vi "AlliGator Export Plugin Parameters to Clipboard.vi"(8 "Error In":errorcluster, 9 "Parameter Names only":bool, 11 "AlliGator IV DVR":refnum<data-value>) -> (0 "Error Out":errorcluster, 1 "Message":string, 3 "AlliGator IV DVR":refnum<data-value>)   [LabVIEW 2021, in "AlliGator Python Plugins.lvlib"]
doc: "Sends a string containing all parameters, internal variables and data accessible to python plugins."
uses:
  AlliGator Python Plugins.lvlib
  AlliGator Internal Variables v2.ctl
  <vilib>/vision/Image Controls.llb/IMAQ Image.ctl
  AlliGator Gate Image Set.ctl
  AlliGator FLI Dataset Type.ctl
  AlliGator Data Series Type.ctl
  AlliGator Dataset Channel.ctl
  AlliGator Gate Arithmetic.ctl
  AlliGator Displayed Image.ctl
  Image/Named ROI Description.ctl
  AlliGator Decay Metadata v3.ctl
  AlliGator Decay Background Subtraction Info.ctl
  AlliGator Baseline Subtraction Method.ctl
  Graphs/XY Graph/XY Graph Plot Shift Parameters.ctl
  Graphs/XY Graph/XY Graph Plot Shift Method.ctl
  AlliGator Decay Extrapolation Parameters.ctl
  Phasor/Calibration Phasor (m, phi).ctl
  Phasor/Phasor Reference Series.ctl
  Phasor/Phasor Calibration Map v2.ctl
  Phasor/Phasor (g, s).ctl
  AlliGator Raw Phasor Plot Data v4.ctl
  Phasor/Phasor Standard Deviation Options.ctl
  AlliGator Phasor Multi-Harmonic Data.ctl
  Phasor/Phasor Harmonic Data.ctl
  AlliGator Decay Fit Options & Parameters v2.ctl
  Fits/IRF(X)PSED/Decay Fit Options v2.ctl
  Fits/Decay Convolution/Decay Model.ctl
  Fits/Residual Type.ctl
  Fits/IRF(X)PSED/Fit Weights Type.ctl
  Fits/Non-linear Fitting Method v2.ctl
  Fits/Fit Calculation Method.ctl
  Fits/Non-linear Fitting Algorithm.ctl
  AlliGator Decay Fit Parameter Constraints 2.ctl
  Fits/IRF(X)PSED/Decay Fit Parameters In List.ctl
  Fits/IRF(X)PSED/MLE Baseline Offset Type.ctl
  AlliGator Decay Preprocessing Parameters.ctl
  Fits/IRF(X)PSED/Decay Fit Parameters & Derived Quantities List.ctl
  ec775fbe-273a-4088-92c5-d89fd97e82c2.vi
  ac933e2b-790f-40e3-b0ca-ca83e507d5bf.vi
  49bf73b8-9f3b-4d7e-9824-64ced49957da.vi
  <userlib>/_OpenG.lib/array/array.llb/Sort 1D Array (String)__ogtk.vi
  <userlib>/_OpenG.lib/array/array.llb/Reorder 1D Array2 (I32)__ogtk.vi
  <vilib>/JDP Science/JSONtext/Variant to JSON Text.vi
  <vilib>/JDP Science/JSONtext/LVClass Serializer/JSONtext LVClass Serializer.lvclass
  AlliGator Settings.lvlib
  Strings/Strings.lvlib
  AlliGator Globals, Variables & Constants.lvlib
  <userlib>/_OpenG.lib/array/array.llb/openg_array.lvlib
  Phasor/Phasor.lvlib
  Image/Image.lvlib
  AlliGator Decay Preprocessing.lvlib
  Graphs/XY Graph/XY Graph Add-Ons.lvlib
  AlliGator Phasor Graph.lvlib
  AlliGator Files.lvlib
  AlliGator Internal Variables.lvlib
  AlliGator Phasor Plot.lvlib
  AlliGator Source Image.lvlib
  Fits/Fits.lvlib
  AlliGator Decay Fit.lvlib
  AlliGator Decay Fit Parameter Map.lvlib
  AlliGator Dual-Channel Datasets.lvlib
panel:
  # "see the AlliGator License on the block diagram (Ctrl+E or Window:Show Block Diagram)"
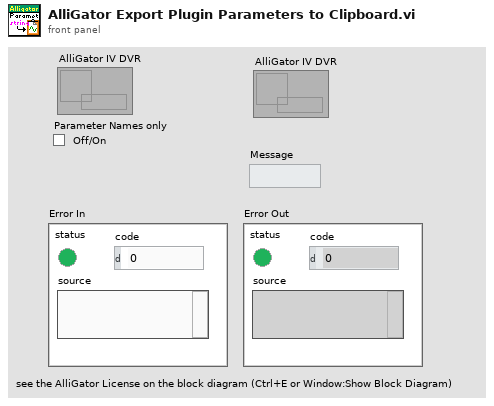
[diagram p1: front panel]
types:
  T1 = typedef "AlliGator Internal Variables.lvlib/AlliGator Internal Variables v2.ctl" = cluster{"Displayed Image":T2, "White Light Image":T2, "Mask Image":T2, "ROI Mask Image":T2, "Current Dataset Images 1":T3, "Background Dataset Images 1":T3, "Current Dataset Images 2":T3, "Background Dataset Images 2":T3, "Current Dataset Arithmetic Images":T3, "Accumulated Dataset Images 1":T3, "Accumulated Dataset Images 2":T3, "Accumulated Dataset Arithmetic Images":T3, "Phasor Plot Image":T2, "Decay Fit Parameter Map Image":T2, "Single Data Point Path":path, "White Light Image Path":path, "Mask Image Path":path, "Time-Series Folder":path, "[Time-Series Paths]":path[], "Current Dataset":i32, "Single Dataset Type":T4, "Current Folder":string, "AlliGator Data Series Type":T5, "# Datasets":i32, "Dual-Channel Dataset":bool, "Selected Channel Name":string, "Dataset Channel":T6, "Channel Arithmetic":T7, "Dual-Channel Background Dataset":bool, "Background Channel":T6, "Dual-Channel Accumulated Dataset":bool, "Start Time":dbl, "[Time-Series Timestamps]":dbl[], "[Intensity Corrections]":dbl[], "Time Series Script":bool, "Type of Displayed Image":T8, "Gate Image Slide":u16, "# Gates":i32, "ROIs":T9[], "ROI Decay":cluster{"t Array":dbl[], "I Array":dbl[]}, "Valid Decay":bool, "Decay  Metadata":T11, "Reference Decay Plot Name":string, "Reference Decay":cluster{"t Array":dbl[], "I Array":dbl[]}, "Decay Shift Plot":cluster{"Time Stamps":dbl[], "Decay Shifts":dbl[]}, "[Decays Max Values]":sgl[], "[Decays Min Values]":sgl[], "Calibration Phasor":T17, "Calibration Phasor Series":T18, "Phasor Calibration Map":T19, "Calibration Map MD5 Digest":string, "Last Raw Phasor":T20, "Last Calibrated Phasor":T20, "Last Calibrated Phasor SDV":T20, "Phasor Graph:Phasor Plot":cluster{"g Array":dbl[], "s Array":dbl[]}, "Phasor Graph:Phasor SDV Plot":cluster{"g Array":dbl[], "s Array":dbl[]}, "[Phasor Graph:Raw Phasor Plots]":T21[], "Phasor Plot locked to Ref 1":i32, "[Phasor Plot(s) locked to Ref 1]":i32[], "[Phasor Plot(s) locked to Ref 2]":i32[], "[Pixel Phasors]":T20[], "[[Sum Image]]":dbl[][], "[[CSG Phasors]]":csg[][], "[[Valid Pixel?]]":bool[][], "I/m/phi Dataset":cluster{"I/m/phi Dataset?":bool, "Base Frequency":dbl[unit], "Harmonic Orders":u8[]}, "Multi Phasor Plot Data":T23, "Decay Fit Options & Parameters":T25, "Fit Options: Decay Preprocessing Parameters":T36, "Fit Options: Reference Decay":cluster{"t Array":dbl[], "I Array":dbl[]}, "Is Full Image Parameters Map":bool, "Is Single-Pixels Parameters Map":bool, "NLSF Parameters Map X Resolution":i32, "NLSF Parameters Map Y Resolution":i32, "[Single Decay Fit Parameters]":dbl[], "Fit Model":T27, "[[Multiple Decays Fit Parameters]]":dbl[][], "[[Multiple Decays Fit Parameter SDVs]]":dbl[][], "[[IRFs]]":dbl[][], "IRF Array Time Axis":dbl[], "Decay Array Time Axis":dbl[], "[Decay Fit Parameter Names]":T37[], "[[Phasor Ratios]]":dbl[][], "[[Average Lifetimes]]":dbl[][], "Amplitude Weighted Average Lifetime":bool, "[Decay Sum]":dbl[], "[[User-defined Quantities]]":dbl[][], "User-defined Quantity":string}
  T2 = typedef "IMAQ Image.ctl" = refnum<image>
  T3 = typedef "AlliGator Internal Variables.lvlib/AlliGator Gate Image Set.ctl" = cluster{"SGL Image Max":T2, "SGL Image Sum":T2, "SGL Gate Images":T2[], "SGL Image Min":T2}
  T4 = typedef "AlliGator Files.lvlib/AlliGator FLI Dataset Type.ctl" = enum16{"HDF5 FLI Dataset", "Gate Image Folder", ".sdt FLI Dataset (Becker & Hickl)", ".ptu FLI Dataset (PicoQuant)", "SS1 FLI Dataset", "SS2 FLI Dataset", "I/m/phi Dataset", ".bin FLI Dataset (PicoQuant Binned)", ".bin FLI Dataset (Piccolo Binned)"}
  T5 = typedef "AlliGator Files.lvlib/AlliGator Data Series Type.ctl" = enum16{"Not a Supported Series", "Gate Images Folder Series", "SwissSPAD 2 Dataset Series", "B&H FLI Dataset Series", "PicoQuant PTU FLI Dataset Series", "PicoQuant BIN FLI Dataset Series", "Piccolo hist BIN FLI Dataset Series", "HDF5 FLI Dataset Series"}
  T6 = typedef "AlliGator Dual-Channel Datasets.lvlib/AlliGator Dataset Channel.ctl" = enum16{"G2", "INT"}
  T7 = typedef "AlliGator Settings.lvlib/AlliGator Gate Arithmetic.ctl" = enum16{"None", "INT-G2", "G2/INT*<INT>", "(1 - G2/INT)*<INT>"}
  T8 = typedef "AlliGator Source Image.lvlib/AlliGator Displayed Image.ctl" = enum16{"Single Gate", "Sum of All Gates", "Max of All Gates", "Min of All Gates", "-", "White Ligth Image", "Mask Image"}
  T9 = typedef "Image.lvlib/Named ROI Description.ctl" = cluster{"ROI Descriptor":T10, "ROI Name":string, "Overlay Color":u32}
  T10 = typedef "ROI Descriptor" = cluster{"Global Rectangle":i32[], "Contours":cluster{"ID":enum32{"External", "Internal"}, "Type":u32, "Coordinates":i32[]}[]}
  T11 = typedef "AlliGator Phasor Graph.lvlib/AlliGator Decay Metadata v3.ctl" = cluster{"ROI Descriptor":T10, "ROI Center":cluster{"X":i32, "Y":i32}, "Decay Background Subtraction Info":T12, "Decay Reverted":bool, "Decay Smoothened":bool, "Decay Straightened":bool, "Fitted Tau (Decay Straightening)":dbl, "Decay Shift Parameters":T14, "Decay Shifted":bool, "Decay Extrapolated":bool, "Decay Extrapolation Parameters":T16, "Decay Normalized":bool, "Fold Decay":bool, "# Folds":u32}
  T12 = typedef "AlliGator Decay Analysis.lvlib/AlliGator Decay Preprocessing.lvlib/AlliGator Decay Background Subtraction Info.ctl" = cluster{"Laser Period":dbl[unit], "Gate Duration":dbl[unit], "Baseline Subtraction Method":T13, "Background Definition Range":cluster{"Min Gate":dbl[unit], "Max Gate":dbl[unit]}, "Total Intensity w/o Bkgd Subtraction":dbl, "Bkgd-subtracted Intensity (exp)":dbl, "# Data Points":i32, "Background/Gate":dbl, "Fitted Lifetime":dbl[unit], "Bkgd-subtracted Intensity (theo)":dbl}
  T13 = typedef "AlliGator Decay Analysis.lvlib/AlliGator Decay Preprocessing.lvlib/AlliGator Baseline Subtraction Method.ctl" = enum16{"Mean", "Min", "Square Gated Single-Exponential", "File", "Constant"}
  T14 = typedef "XY Graph Add-Ons.lvlib/XY Graph Plot Shift Parameters.ctl" = cluster{"Type":T15, "Shift":dbl[unit], "Threshold":dbl, "Rotate":bool}
  T15 = typedef "XY Graph Add-Ons.lvlib/XY Graph Plot Shift Method.ctl" = enum16{"Default", "CFD", "Threshold", "Cross-Correlation"}
  T16 = typedef "AlliGator Decay Analysis.lvlib/AlliGator Decay Preprocessing.lvlib/AlliGator Decay Extrapolation Parameters.ctl" = cluster{"Additional Points":u32, "Head Fraction":dbl, "Fitted Tau":dbl, "Use Periodicity":bool, "Use Cursors":bool, "Tail Fraction":dbl}
  T17 = typedef "Phasor.lvlib/Calibration Phasor (m, phi).ctl" = cluster{"m":dbl, "phi":dbl, "Phasor Frequency":dbl[unit], "Reference Lifetime":dbl[unit]}
  T18 = typedef "Phasor.lvlib/Phasor Reference Series.ctl" = cluster{"m Array":dbl[], "phi Array":dbl[], "Phasor Frequency":dbl[unit], "Calibration Lifetime":dbl[unit]}
  T19 = typedef "Phasor.lvlib/Phasor Calibration Map v2.ctl" = cluster{"Phasor Frequency":dbl[unit], "Calibration Lifetime":dbl[unit], "ROI Centers":cluster{"X":i32, "Y":i32}[], "ROI Descriptors":T10[], "Map Resolution X":i32, "Map Resolution Y":i32, "z Array":cdb[]}
  T20 = typedef "Phasor.lvlib/Phasor (g, s).ctl" = cluster{"g":dbl, "s":dbl}
  T21 = typedef "AlliGator Phasor Graph.lvlib/AlliGator Raw Phasor Plot Data v4.ctl" = cluster{"Phasor Plot Name":string, "Raw Phasor Plot":T20[], "Phasor Frequency":dbl[unit], "[Decay Metadata]":T11[], "Raw Phasor Plot SDV":T20[], "Phasor SDV Options":T22, "[Calibration Phasor]":T17[]}
  T22 = typedef "Phasor.lvlib/Phasor Standard Deviation Options.ctl" = cluster{"Compute Estimated SDV":bool, "# Replicas":u32, "Use Estimated Average Phasor":bool}
  T23 = typedef "AlliGator Phasor Plot.lvlib/AlliGator Phasor Multi-Harmonic Data.ctl" = cluster{"Base Frequency":dbl[unit], "# Harmonics":u8, "Harmonic Orders":u8[], "Phasor Plot Settings Checksum":u64, "Phasor Harmonic Data Array":T24[]}
  T24 = typedef "Phasor.lvlib/Phasor Harmonic Data.ctl" = cluster{"Phasor Harmonic Name":string, "Phasor Plot Settings Checksum":u64, "Phasor Frequency":dbl[unit], "Base Frequency":dbl[unit], "Harmonic Order":u8, "Phasor Plot Parameters":string, "Phasor Array [[CSG]]":csg[][], "Dataset File Path":path}
  T25 = typedef "AlliGator Decay Fit Parameter Map.lvlib/AlliGator Decay Fit Options & Parameters v2.ctl" = cluster{"SYNC Period":dbl[unit], "Fit Options":T26, "Fit Parameter Constraints":T33[], "MLE Baseline Offset":dbl, "MLE Baseline Offset Type":T35}
  T26 = typedef "Fits.lvlib/Decay Fit Options v2.ctl" = cluster{"Show Fit Residuals":bool, "Fit Model":T27, "Residual Type":T28, "Max Decay Percentile":dbl, "Min Decay Percentile":dbl, "Show Full Decay":bool, "Weights":T29, "Fitting Method":T30, "Compute Parameter Uncertainties":bool, "Periodic Boundaries":bool, "Model Calculation":T31, "Period":dbl[unit], "Termination Criteria":cluster{"Max Iterations":i32, "Max Function Calls":i32, "Max Time":dbl[unit], "Function Tolerance":dbl, "Parameter Tolerance":dbl, "Gradient Tolerance":dbl, "Min Lambda":dbl, "Max Lambda":dbl, "Initial Tick Count":u32}, "Offset Resolution":dbl[unit], "Use Local IRF":bool, "Fitting Algorithm":T32}
  T27 = typedef "Fits.lvlib/Decay Model.ctl" = enum16{"1-Exponential", "2-Exponentials"}
  T28 = typedef "Fits.lvlib/Residual Type.ctl" = enum16{"Standard", "Normalized", "Reduced"}
  T29 = typedef "Fits.lvlib/Fit Weights Type.ctl" = enum16{"Unweighted", "1/Variance", "Best of All"}
  T30 = typedef "Fits.lvlib/Non-linear Fitting Method v2.ctl" = enum16{"Least Square", "Least Absolute Residual", "Bisquare", "MLE", "-", "Best of All"}
  T31 = typedef "Fits.lvlib/Fit Calculation Method.ctl" = enum16{"Simulation", "Convolution", "Integration"}
  T32 = typedef "Fits.lvlib/Non-linear Fitting Algorithm.ctl" = enum16{"Levenberg-Marquardt", "Trust-Region Dogleg"}
  T33 = typedef "AlliGator Decay Analysis.lvlib/AlliGator Decay Fit.lvlib/AlliGator Decay Fit Parameter Constraints 2.ctl" = cluster{"Fit Parameter":T34, "Min Value":dbl, "Max Value":dbl, "Global":bool, "Used":bool}
  T34 = typedef "Fits.lvlib/Decay Fit Parameters In List.ctl" = enum16{"Offset", "Baseline", "A_1", "tau_1", "A_2", "tau_2"}
  T35 = typedef "Fits.lvlib/MLE Baseline Offset Type.ctl" = enum32{"Absolute", "Percentage"}
  T36 = typedef "AlliGator Decay Analysis.lvlib/AlliGator Decay Preprocessing.lvlib/AlliGator Decay Preprocessing Parameters.ctl" = cluster{"Background Subtraction":bool, "Straighten Decay":bool, "Reverse Gates":bool, "1-Normalized Decay":bool, "Smoothen Decay":bool, "Smoothing Parameter":dbl, "Shift Decay":bool, "Decay Shift Parameters":T14, "Extrapolate Decay":bool, "Additional Points":u32, "Head Fraction":dbl, "Pixel-Normalize Decay":bool, "Use Periodicity":bool, "Use Cursors":bool, "Tail Fraction":dbl, "Use Decay Pre-Processing":bool, "Fold Decay":bool, "# Folds":u32, "[0-1]-Normalized Decay":bool}
  T37 = typedef "Fits.lvlib/Decay Fit Parameters & Derived Quantities List.ctl" = enum16{"Offset", "Baseline", "A_1", "tau_1", "A_2", "tau_2", "<tau>_a", "f1_a", "f2_a", "<tau>_i", "f1_i", "f2_i", "-", "R^2", "Chi^2"}
  T38 = typedef "AlliGator Settings.lvlib/AlliGator Settings List.ctl" = enum16{"GUI:Visible Settings Tab", "GUI:Last Run Version", "Source Image:Use Image Histogram for Contrast", "Source Image:Low Count Pixels Rejection Options", "Source Image:High Count Pixels Rejection Options", "Source Image:Use Image Brightness", "Source Image:Blend Overlay with Image Background", "Source Image:Use Fixed ROI Diameter", "Source Image:ROI Diameter", "Source Image:ROI Center Color", "Source Image:Peak Threshold", "Source Image:Intensity Threshold", "Source Image:Image Binning Options", "Source Image:Image Smoothing Options", "Source Image:Image Histogram Active", "Source Image:Invert Binary Mask", "Source Image:Hot Pixel Removal", "Source Image:Overlay Analyzed ROI Center", "Source Image:Auto-Adjust Contrast", "Source Image:Histogram Lower Percentile", "Source Image:Histogram Upper Percentile", "Source Image:Save Source Image", "Source Image:Scale Bar Options", "Source Image:Image Resolution (Pixel Size)", "Source Image:Flatfield Correction", "Source Image:Show Dead Left Columns Correction", "Source Image:Dead Left Columns Correction", "Source Image:Image Pre-Processing Operations Order", "Data Information:Gate Width", "Data Information:Nanotime Gate Separation", "Data Information:Macrotime Gate Separation", "Data Information:Gate Step", "Data Information:# Gates", "Data Information:Gate Image Exposure", "Data Information:Gate Image Integration", "Data Information:Gates to Skip", "Data Information:Gates to Keep", "Data Information:Define Gates to", "Data Information:Channel Name", "Data Information:Available Channel Names", "Data Information:Channel Arithmetic", "Data Information:Background File Subtraction", "Data Information:Background File", "Data Information:Background Scaling Factor", "Data Information:Background Pile-up Correction", "Data Information:Background Pixel Well Capacity", "Data Information:Laser Period", "Data Information:SYNC Period", "Data Information:Pile-up Correction", "Data Information:Pixel Well Capacity", "Data Information:Dataset Scaling Factor", "Fluorescence Decay_Decay Pre-Processing:Reverse Gates", "Fluorescence Decay_Decay Pre-Processing:Verbose Decay Pre-Processing", "Fluorescence Decay_Decay Pre-Processing:Use Decay Pre-Processing", "Fluorescence Decay_Decay Pre-Processing:Background Subtraction", "Fluorescence Decay_Decay Pre-Processing:Background Definition Range", "Fluorescence Decay_Decay Pre-Processing:Baseline Subtraction Method", "Fluorescence Decay_Decay Pre-Processing:Decay Pre-Processing Operations Order", "Fluorescence Decay_Decay Pre-Processing:Smoothing Parameter", "Fluorescence Decay_Decay Pre-Processing:Shift Decay", "Fluorescence Decay_Decay Pre-Processing:Decay Shift Parameters", "Fluorescence Decay_Decay Pre-Processing:Fold Decay", "Fluorescence Decay_Decay Pre-Processing:# Folds", "Fluorescence Decay_Decay Pre-Processing:1-Normalize Decay", "Fluorescence Decay_Decay Pre-Processing:[0-1]-Normalize Decay", "Fluorescence Decay_Decay Pre-Processing:Smoothen Decay", "Fluorescence Decay_Decay Pre-Processing:Extrapolate Decay", "Fluorescence Decay_Decay Pre-Processing:Use Periodicity", "Fluorescence Decay_Decay Pre-Processing:Use Cursors", "Fluorescence Decay_Decay Pre-Processing:Tail Fraction", "Fluorescence Decay_Decay Pre-Processing:Head Fraction", "Fluorescence Decay_Decay Pre-Processing:Additional Points", "Fluorescence Decay_Decay Pre-Processing:Straighten Decay", "Fluorescence Decay_Decay Pre-Processing:Constant Background", "Fluorescence Decay_Decay Pre-Processing:Pixel-Normalize Decay", "Fluorescence Decay_Advanced Analysis:Extract IRF instead of Decay", "Fluorescence Decay_Advanced Analysis:IRF Extraction Options", "Fluorescence Decay_Advanced Analysis:IRF Optimization Options", "Fluorescence Decay_Advanced Analysis:Square Pulse Options", "Fluorescence Decay_Advanced Analysis:IRF Order", "Fluorescence Decay_Advanced Analysis:IRF Time Constants", "Fluorescence Decay_Advanced Analysis:Wavelet Analysis Options", "Fluorescence Decay_Advanced Analysis:Average Lifetime Options", "Fluorescence Decay_Fit Options:Fit Options", "Fluorescence Decay_Fit Options:Use Legacy Fitting Approach", "Fluorescence Decay_Fit Options:Use Data Information Laser Period", "Fluorescence Decay_Fit Parameters:Displayed Fit Parameters", "Fluorescence Decay_Fit Parameters:Fit Parameter Constraints", "Fluorescence Decay_Fit Parameters:Export Tabulated Results", "Fluorescence Decay_Fit Parameters:MLE Baseline Offset Type", "Fluorescence Decay_Fit Parameters:MLE Baseline Offset", "Fluorescence Decay_Fit Parameters:Guess Parameter Names", "Fluorescence Decay_Fit Parameters:Guess Parameter Values", "Fluorescence Decay_Fit Parameters:Guess Parameters Options", "Fluorescence Decay_Styles:Show Last Decay Only", "Fluorescence Decay_Styles:Decay Graph Color Array", "Fluorescence Decay:Decay Graph Active", "Fluorescence Decay Statistics:Min Peak Value", "Fluorescence Decay Statistics:Reject Low Decay Peak Pixels", "Fluorescence Decay Statistics:Reject High Decay Peak Pixels", "Fluorescence Decay Statistics:Max Peak Value", "Time Traces:Use File Timestamp", "Time Traces:Time Step", "Time Traces:Use Intensity Correction File", "Time Traces:Intensity Correction File", "Phasor Plot:Phasor Plot Smoothing Options", "Phasor Plot:Phasor Plot Size", "Phasor Plot:Phasor Plot Graphics Options", "Phasor Plot:Cumulative Phasor Plot", "Phasor Plot:Use Phasor Brightness", "Phasor Plot:Blend Overlay with Phasor Background", "Phasor Plot:Save Phasor Plot", "Phasor Plot:Show References", "Phasor Plot:Phasor Ratio Decay Range", "Phasor Plot:Exponential Fading", "Phasor Plot:Phasor Ratio Reference Colors", "Phasor Plot:Reference Radius", "Phasor Plot:Show Color Map Vertices", "Phasor Plot:Phasor Plot Active", "Phasor Plot:Phasor Ratio Color Map Type", "Phasor Plot:Phasor Ratio Color Map", "Phasor Plot:Phasor Ratio Display Range", "Phasor Plot:Selected Image ROI(s)", "Phasor Plot:All Image ROIs", "Phasor Plot:Selected Phasor Plot ROI(s)", "Phasor Plot:All Phasor Plot ROIs", "Phasor Plot:Phasor Ratio Color-Coded Quantity", "Phasor Plot:Store Phasor Harmonics", "Phasor Plot:Draw Reference Segment", "Phasor Plot:User-Defined Quantity", "Phasor Graph:Phasor Frequency", "Phasor Graph:Phasor Ratio Type", "Phasor Graph:Pixel-level Phasor Computation", "Phasor Graph:Save Phasor Graph", "Phasor Graph:Phasor Graph Active", "Phasor Graph:Phasor SDV Options", "Phasor Calibration:Use Backup Calibration if needed", "Phasor Graph:Define Shortest Lifetime as", "Phasor Calibration:Backup Calibration Type", "Phasor Calibration:Calibration Type", "Phasor Calibration:Calibration Lifetime", "Phasor Calibration:Calibration Map Algorithm", "Single-Exponential Phasor Locus (SEPL):Gate Parameters", "Single-Exponential Phasor Locus (SEPL):User-defined Gate", "Single-Exponential Phasor Locus (SEPL):User-defined IRF", "Single-Exponential Phasor Locus (SEPL):Phasor Parameters", "Single-Exponential Phasor Locus (SEPL):Decay & IRF Parameters", "Single-Exponential Phasor Locus (SEPL):Display Parameters", "Lifetime Analysis:Decay Analysis Parameters", "Lifetime Analysis:Lifetime Map Active", "Plugins:Python Settings", "Miscellaneous:Verbose Mode", "Miscellaneous:Beep after Script", "Miscellaneous:Saved Image File Format", "Miscellaneous:Exported Gate Image Settings", "Miscellaneous:Include Loading in Timing", "Miscellaneous:Verbose Settings Mode", "Miscellaneous:Histogram Options", "Miscellaneous:Beep on Error", "Miscellaneous:# Logical Processors Used", "Miscellaneous:ROI Description Max Characters", "Miscellaneous:Verbose Error Mode", "Miscellaneous:Transparent Mask Color"}
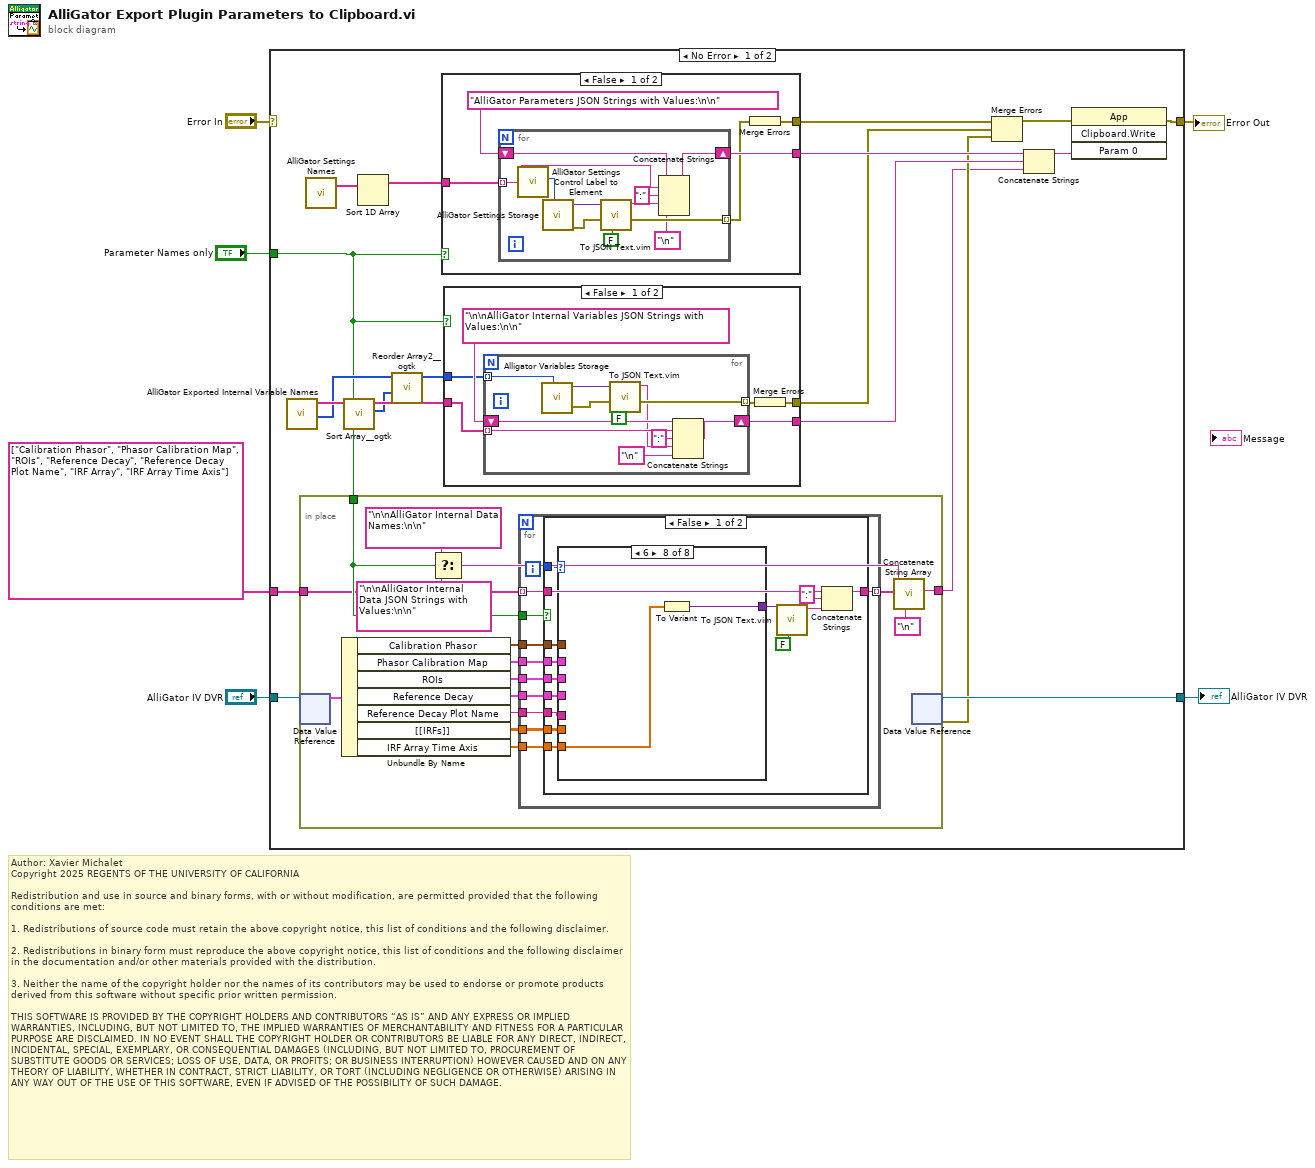
[diagram p0: block diagram]
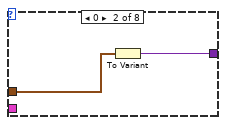
[diagram p3: hidden frame]
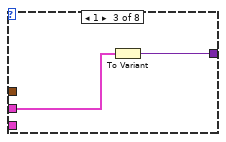
[diagram p4: hidden frame]
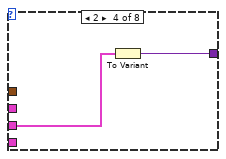
[diagram p5: hidden frame]
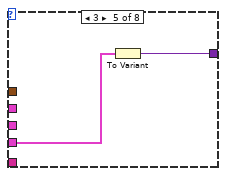
[diagram p6: hidden frame]
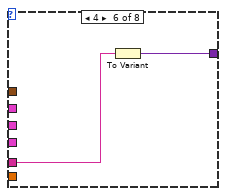
[diagram p7: hidden frame]
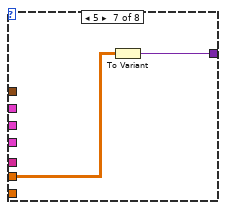
[diagram p8: hidden frame]
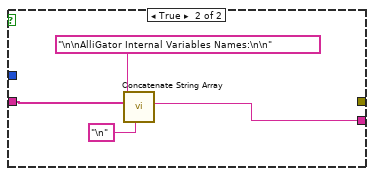
[diagram p10: hidden frame]
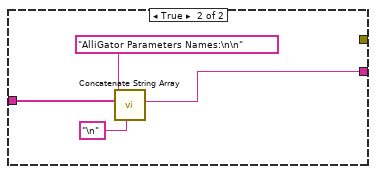
[diagram p11: hidden frame]
diagram:
  # "Author: Xavier Michalet\nCopyright 2025 REGENTS OF THE UNIVERSITY OF CALIFORNIA\n\nRedistribution and use in source and binary forms, with or without modification, are permitted provided that the following conditions are met:\n\n1. Redistributions of source code must retain the above copyright notice, this list of conditions and the following disclaimer.\n\n2. Redistributions in binary form must reproduce the above copyright notice, this list of conditions and the following disclaimer in the documentation and/or other materials provided with the distribution.\n\n3. Neither the name of the copyright holder nor the names of its contributors may be used to endorse or promote products derived from this software without specific prior written permission.\n\nTHIS SOFTWARE IS PROVIDED BY THE COPYRIGHT HOLDERS AND CONTRIBUTORS “AS IS” AND ANY EXPRESS OR IMPLIED WARRANTIES, INCLUDING, BUT NOT LIMITED TO, THE IMPLIED WARRANTIES OF MERCHANTABILITY AND FITNESS FOR A PARTICULAR PURPOSE ARE DISCLAIMED. IN NO EVENT SHALL THE COPYRIGHT HOLDER OR CONTRIBUTORS BE LIABLE FOR ANY DIRECT, INDIRECT, INCIDENTAL, SPECIAL, EXEMPLARY, OR CONSEQUENTIAL DAMAGES (INCLUDING, BUT NOT LIMITED TO, PROCUREMENT OF SUBSTITUTE GOODS OR SERVICES; LOSS OF USE, DATA, OR PROFITS; OR BUSINESS INTERRUPTION) HOWEVER CAUSED AND ON ANY THEORY OF LIABILITY, WHETHER IN CONTRACT, STRICT LIABILITY, OR TORT (INCLUDING NEGLIGENCE OR OTHERWISE) ARISING IN ANY WAY OUT OF THE USE OF THIS SOFTWARE, EVEN IF ADVISED OF THE POSSIBILITY OF SUCH DAMAGE."
  n1 = case shown="No Error" "Error In" {
    selector: "Error In" -> [_ w125]
    tunnel: "Parameter Names only" -> [w11 _]
    tunnel: [w15 w125] -> w5
    tunnel: "AlliGator IV DVR" -> [w14 w124]
    tunnel: [w13 w124] -> w2
    tunnel: string[] ["Calibration Phasor", "Phasor Calibration Map", "ROIs", "Reference Decay", "Reference Decay Plot Name", "IRF Array", "IRF Array Time Axis"] ("<JSON>") -> [w10 _]
    frame No Error {
      n2 = call "AlliGator Exported Internal Variable Names.vi"() -> ("Indices of Exported IVs"=w19:i32[], "Exported IV Name Array"=w24:string[])  [unwired: 10 in]
      n3 = in-place {
        in-place-border: w11 -> [w41]
        in-place-border: w10 -> [w40]
        in-place-border: [w39] -> w9
        n4 = in-place-dvr #1(w14) -> (w42:T1)  [unwired: 1 out]
        n5 = Unbundle By Name(w42) -> ("Calibration Phasor"=w38:T17, "Phasor Calibration Map"=w37:T19, "ROIs"=w36:T9[], "Reference Decay"=w35:cluster{"t Array":dbl[], "I Array":dbl[]}, "Reference Decay Plot Name"=w34:string, "[[IRFs]]"=w33:dbl[][], "IRF Array Time Axis"=w32:dbl[])
        n6 = Select(t="\n\nAlliGator Internal Data Names:\n\n", s=w41, f="\n\nAlliGator Internal Data JSON Strings with Values:\n\n") -> (s? t:f=w28:string)
        n7 = for {
          tunnel: w38 -> [w53]
          tunnel: w37 -> [w52]
          tunnel: w36 -> [w51]
          tunnel: w35 -> [w50]
          tunnel: w34 -> [w49]
          tunnel: w33 -> [w48]
          tunnel: w32 -> [w47]
          tunnel: [w46] -> w31 mode=indexing
          tunnel: w41 -> [w45]
          tunnel: w40 -> [w44] mode=indexing
          i -> [w43]
          n8 = case shown="False" w45 {
            tunnel: w53 -> [w67 _]
            tunnel: w52 -> [w66 _]
            tunnel: w51 -> [w65 _]
            tunnel: w50 -> [w64 _]
            tunnel: w49 -> [w63 _]
            tunnel: w48 -> [w62 _]
            tunnel: w47 -> [w61 _]
            tunnel: [w54 w82] -> w46
            tunnel: w44 -> [w56 w82]
            tunnel: w43 -> [w59 _]
            frame False {
              n9 = case shown="6" w59 {
                tunnel: w67 -> [_ w69 _ _ _ _ _ _]
                tunnel: w66 -> [_ _ w70 _ _ _ _ _]
                tunnel: w65 -> [_ _ _ w72 _ _ _ _]
                tunnel: w64 -> [_ _ _ _ w74 _ _ _]
                tunnel: w63 -> [_ _ _ _ _ w76 _ _]
                tunnel: w62 -> [_ _ _ _ _ _ w78 _]
                tunnel: w61 -> [_ _ _ _ _ _ _ w80]
                tunnel: [_ w68 w71 w73 w75 w77 w79 w81] -> w60
                frame -1, Default {
                }
                frame 0 {
                  n10 = To Variant(anything=w69) -> (Variant=w68:variant)
                }
                frame 1 {
                  n11 = To Variant(anything=w70) -> (Variant=w71:variant)
                }
                frame 2 {
                  n12 = To Variant(anything=w72) -> (Variant=w73:variant)
                }
                frame 3 {
                  n13 = To Variant(anything=w74) -> (Variant=w75:variant)
                }
                frame 4 {
                  n14 = To Variant(anything=w76) -> (Variant=w77:variant)
                }
                frame 5 {
                  n15 = To Variant(anything=w78) -> (Variant=w79:variant)
                }
                frame 6 {
                  n16 = To Variant(anything=w80) -> (Variant=w81:variant)
                }
              }
              n17 = call "To JSON Text.vim"("Pretty Print?"=FALSE, "Anything"=w60) -> ("<JSON>"=w57:string)  [unwired: 8 in, 1 out]
              n18 = Concatenate Strings(w56, ":" ("string"), w57) -> (w54:string)
            }
            frame True {
            }
          }
        }
        n19 = call "Concatenate String Array.vi"("Separator (TAB)"="\n", "String Array"=w31, "Prefix (\"\")"=w28) -> ("Formatted String"=w39:string)  [unwired: 8 in]
        n20 = in-place-dvr #1() -> (w13:refnum<data-value>, w12:errorcluster)  [unwired: 1 in]
      }
      n21 = call "AlliGator Settings Names.vi"() -> ("Settings Name Array"=w8:string[])  [unwired: 2 in, 1 out]
      n22 = call-poly <userlib>:"Sort Array__ogtk.vi"("Array in"=w24) -> ("Sorted Pointers"=w20:i32[], "Sorted Array out"=w23:string[])  [unwired: 9 in]
      n23 = Sort 1D Array(array=w8) -> (sorted array=w7:string[])
      n24 = call-poly <userlib>:"Reorder Array2__ogtk.vi"("indices"=w20, "array"=w19) -> ("reordered array"=w18:i32[])  [unwired: 9 in]
      n25 = case shown="False" w11 {
        tunnel: w7 -> [w108 w123]
        tunnel: [w107 w121] -> w25
        tunnel: [w105 _] -> w26
        frame False {
          n26 = for {
            tunnel: w108 -> [w111] mode=indexing
            shift-right: [w109] -> w107
            shift-left: "AlliGator Parameters JSON Strings with Values:\n\n" -> [w110]
            tunnel: [w113] -> w106 mode=indexing
            n27 = call "AlliGator Settings Control Label to Element.vi"("Control Label"=w111) -> ("AlliGator Settings List Element"=w119:T38)  [unwired: 7 in, 1 out]
            n28 = call "AlliGator Settings Storage.vi"("AlliGator Settings List"=w119) -> ("Error Out"=w117:errorcluster, "Variant Data out"=w118:variant)  [unwired: 9 in]
            n29 = call "To JSON Text.vim"("Pretty Print?"=FALSE, "error in (no error)"=w117, "Anything"=w118) -> ("error out"=w113:errorcluster, "<JSON>"=w115:string)  [unwired: 7 in]
            n30 = Concatenate Strings(w110, w111, ":" ("string"), w115, "\n" ("string")) -> (w109:string)
          }
          n31 = Merge Errors(w106) -> (w105:errorcluster)
        }
        frame True {
          n32 = call "Concatenate String Array.vi"("Separator (TAB)"="\n", "String Array"=w123, "Prefix (\"\")"="AlliGator Parameters Names:\n\n") -> ("Formatted String"=w121:string)  [unwired: 8 in]
        }
      }
      n33 = case shown="False" w11 {
        tunnel: w23 -> [w88 w102]
        tunnel: [w86 w100] -> w21
        tunnel: w18 -> [w85 _]
        tunnel: [w83 _] -> w16
        frame False {
          n34 = for {
            tunnel: w88 -> [w91] mode=indexing
            shift-right: [w92] -> w86
            shift-left: "\n\nAlliGator Internal Variables JSON Strings with Values:\n\n" -> [w93]
            tunnel: w85 -> [w99] mode=indexing
            tunnel: [w96] -> w84 mode=indexing
            n35 = call "Alligator Variables Storage.vi"("AlliGator Variable"=w99) -> ("Error Out"=w97:errorcluster, "Data out"=w98:variant)  [unwired: 8 in, 1 out]
            n36 = call "To JSON Text.vim"("Pretty Print?"=FALSE, "error in (no error)"=w97, "Anything"=w98) -> ("error out"=w96:errorcluster, "<JSON>"=w90:string)  [unwired: 7 in]
            n37 = Concatenate Strings(w93, w91, ":" ("string"), w90, "\n" ("string")) -> (w92:string)
          }
          n38 = Merge Errors(w84) -> (w83:errorcluster)
        }
        frame True {
          n39 = call "Concatenate String Array.vi"("Separator (TAB)"="\n", "String Array"=w102, "Prefix (\"\")"="\n\nAlliGator Internal Variables Names:\n\n") -> ("Formatted String"=w100:string)  [unwired: 8 in]
        }
      }
      n40 = Merge Errors(w26, w16, w12) -> (w17:errorcluster)
      n41 = Concatenate Strings(w25, w21, w9) -> (w22:string)
      n42 = invoke class="App" method="Clipboard.Write"(error in=w17, "Param 0"=w22) -> (error out=w15:errorcluster)  [unwired: 2 in, 3 out]
    }
    frame Error {
    }
  }
  "Error Out" <- w5
  "AlliGator IV DVR" <- w2
